vi "Fix Data Files.vi"() -> ()   [LabVIEW 2017]
panel:
  out "result string":string
  out "String":string
  in  "Path":path=path "D:/Crabtree_backup/Crabtree/Crabtree LAB Panel/Lab Panel V2/Data/B"
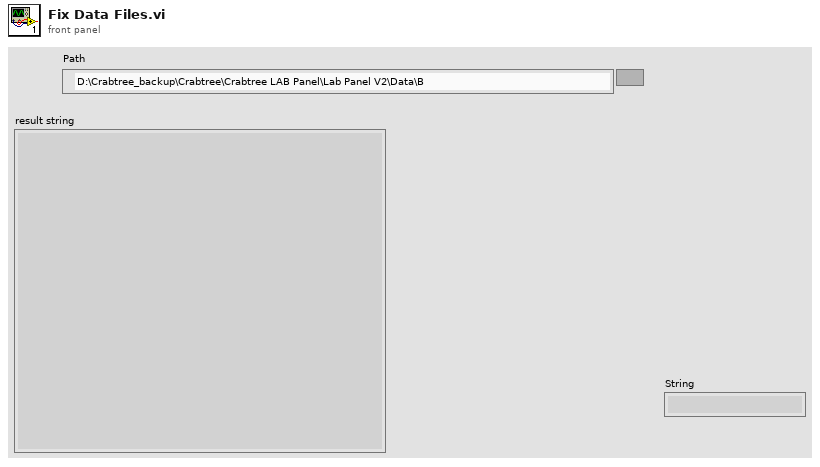
[diagram p1: front panel]
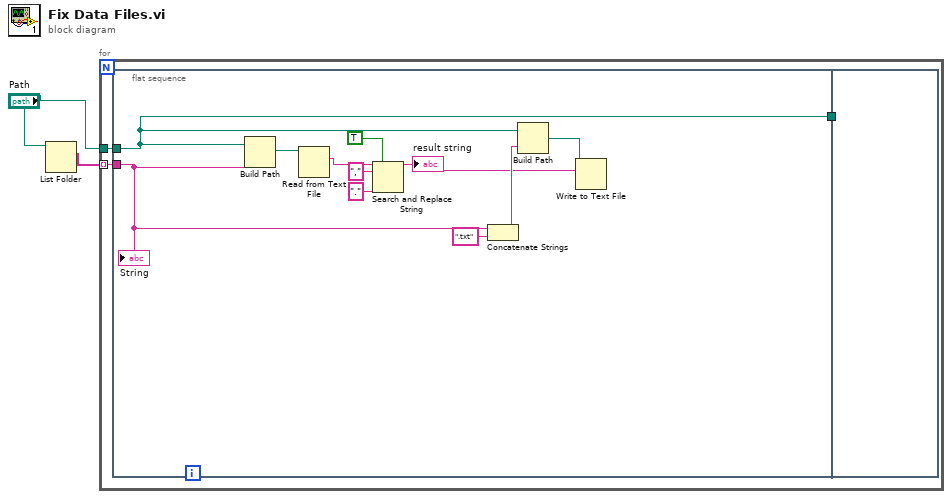
[diagram p0: block diagram]
diagram:
  n1 = List Folder(path="Path") -> (filenames=w1:string[])  [unwired: 3 in, 3 out]
  n2 = for {
    tunnel: "Path" -> [w5]
    tunnel: w1 -> [w4] mode=indexing
    n3 = flat-sequence {
      tunnel: w5 -> [w6]
      tunnel: w4 -> [w11]
      tunnel: [w6] -> w3
      tunnel: w3 -> [_]
      frame #0 {
        n4 = Build Path(base path=w6, name or relative path=w11) -> (appended path=w16:path)
        n5 = Read from Text File(file (use dialog)=w16) -> (text=w15:string)  [unwired: 3 in, 3 out]
        n6 = Search and Replace String(replace all?=TRUE ("replace all? (F)"), input string=w15, search string=",", replace string="." ("replace string (\"\")")) -> (result string=w8:string)  [unwired: 4 in, 3 out]
        "result string" <- w8
        n7 = Concatenate Strings(w11, ".txt" ("string")) -> (w10:string)
        n8 = Build Path(base path=w6, name or relative path=w10) -> (appended path=w9:path)
        n9 = Write to Text File(file (use dialog)=w9, text=w8) -> ()  [unwired: 2 in, 3 out]
        "String" <- w11
      }
      frame #1 {
      }
    }
  }
